vi "Get Input Parameter.vi"(8 "error in (no error)":errorcluster, 10 "Control Name":string, 11 "Parametric VI Call In":refnum<class "Parametric VI Call.lvclass">) -> (0 "error out":errorcluster, 2 "Value":variant)   [LabVIEW 2020, in "Parametric VI Call.lvclass"]
uses:
  Parametric VI Call.lvclass
  Parametric VI Call.lvclass/Parametric VI Call.ctl
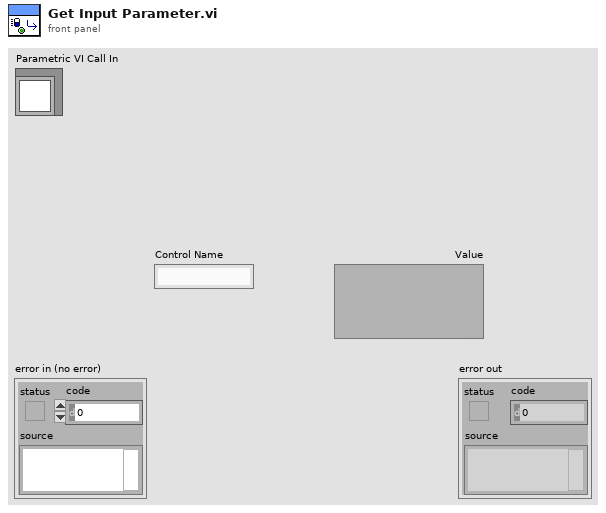
[diagram p1: front panel]
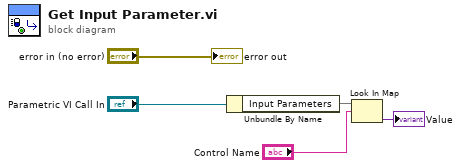
[diagram p0: block diagram]
diagram:
  n1 = Unbundle By Name("Parametric VI Call In") -> ("Input Parameters"=w5:map{string, variant})
  n2 = Look In Map(map=w5, key="Control Name") -> (value=→"Value":variant)  [unwired: 1 in, 1 out]
  "error out" <- "error in (no error)"
